vi "Load Temp.vi"(8 "error in (no error)":errorcluster, 10 "temp file name":string="ic_sparc.cfg", 11 "Channel in":refnum<class "Channel.lvclass">) -> (0 "error out":errorcluster, 3 "Channel out":refnum<class "Channel.lvclass">)   [LabVIEW 2018, in "Channel.lvclass"]
uses:
  Channel.lvclass
  Channel.lvclass/Channel.ctl
  <vilib>/Utility/config.llb/Read Key (String).vi
  Interface/Interface.lvclass
  <vilib>/Utility/config.llb/NI_LVConfig.lvlib
panel:
  in  "Temp cluster":T1={"COOLER_POWER_STATUS"=0, "CURRENT_TEMPERATURE"=20} {"CURRENT_TEMPERATURE" min=0 max=0; "COOLER_POWER_STATUS" items=["Cooler OFF", "Cooler ON"]}
  out "file created?":bool
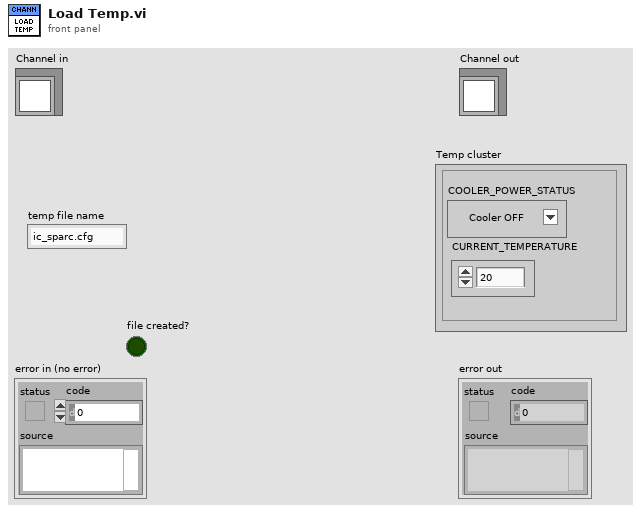
[diagram p1: front panel]
types:
  T1 = cluster{"COOLER_POWER_STATUS":i16, "CURRENT_TEMPERATURE":i8}
  T2 = typedef "NI_LVConfig.lvlib/Config Data RefNum.ctl" = refnum<k1>
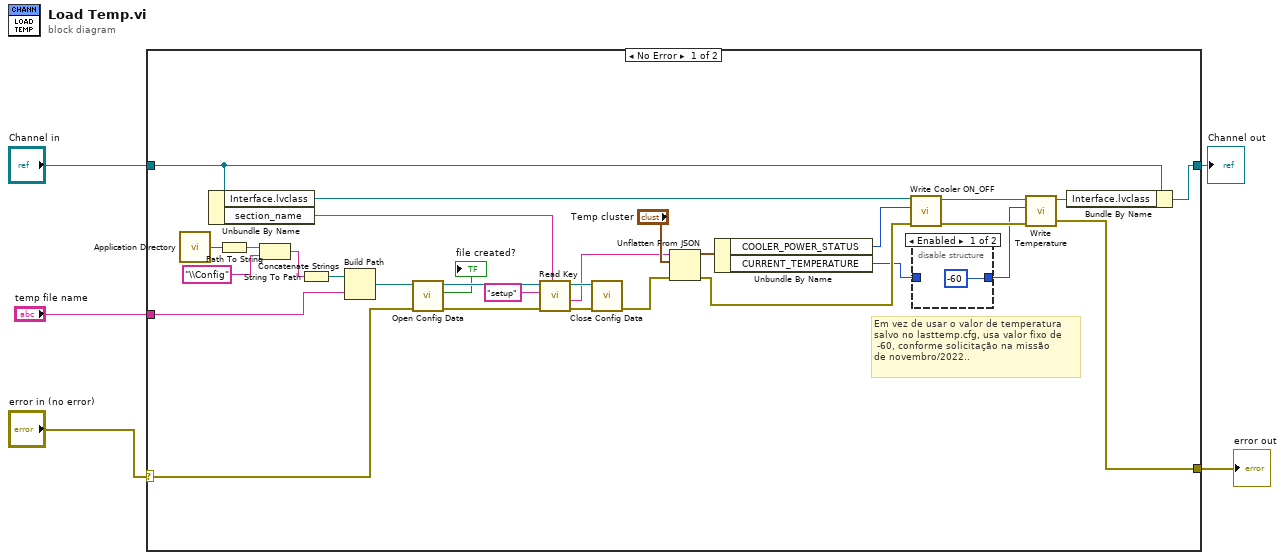
[diagram p0: block diagram]
diagram:
  n1 = case shown="No Error" "error in (no error)" {
    selector: "error in (no error)" -> [w29 w39]
    tunnel: [w10 w39] -> w1
    tunnel: [w30 w38] -> w2
    tunnel: "Channel in" -> [w31 w38]
    tunnel: "temp file name" -> [w24 _]
    frame No Error {
      # "Em vez de usar o valor de temperatura \nsalvo no lasttemp.cfg, usa valor fixo de\n -60, conforme solicitação na missão \nde novembro/2022.."
      n2 = call <vilib>:"Application Directory.vi"() -> ("Application Directory"=w23:path)
      n3 = Unbundle By Name(w31) -> ("Interface.lvclass"=w18:refnum<class "Interface.lvclass">, "section_name"=w34:string)
      n4 = Path To String(path=w23) -> (string=w22:string)
      n5 = Concatenate Strings(w22, "\\Config" ("string")) -> (w20:string)
      n6 = String To Path(string=w20) -> (path=w19:path)
      n7 = Build Path(base path=w19, name or relative path=w24) -> (appended path=w35:path)
      n8 = call <vilib>:"Open Config Data.vi"("error in (no error)"=w29, "configuration file path"=w35) -> ("error out"=w28:errorcluster, "file created?"=→"file created?":bool, "refnum"=w33:T2)  [unwired: 7 in]
      n9 = call-poly <vilib>:"Read Key.vi"("section"=w34, "error in (no error)"=w28, "key"="setup", "refnum"=w33) -> ("error out"=w25:errorcluster, "value"=w16:string, "refnum out"=w26:T2)  [unwired: 4 in, 1 out]
      n10 = call <vilib>:"Close Config Data.vi"("error in (no error)"=w25, "refnum"=w26) -> ("error out"=w9:errorcluster)  [unwired: 8 in, 1 out]
      n11 = Unflatten From JSON(JSON string=w16, type and defaults="Temp cluster", error in (no error)=w9) -> (value=w15:T1, error out=w8:errorcluster)  [unwired: 4 in]
      n12 = Unbundle By Name(w15) -> ("COOLER_POWER_STATUS"=w14:i16, "CURRENT_TEMPERATURE"=w6:i8)
      n13 = call-dynamic "Write Cooler ON_OFF.vi"("error in (no error)"=w8, "Cooler ON/OFF"=w14, "Interface in"=w18) -> ("error out"=w11:errorcluster, "Interface out"=w13:refnum<class "Interface.lvclass">)  [unwired: 7 in]
      n14 = disable-structure shown="Enabled" {
        disable-tunnel: [i8 -60 w37] -> w7
        disable-tunnel: w6 -> [_ w37]
        frame Enabled {
        }
        frame Disabled {
        }
      }
      n15 = call-dynamic "Write Temperature.vi"("error in (no error)"=w11, "Temperature"=w7, "Interface in"=w13) -> ("error out"=w10:errorcluster, "Interface out"=w12:refnum<class "Interface.lvclass">)  [unwired: 7 in]
      n16 = Bundle By Name(cluster=w31, "Interface.lvclass"=w12) -> (w30:refnum<class "Channel.lvclass">)
    }
    frame Error {
    }
  }
  "error out" <- w1
  "Channel out" <- w2
